vi "altera_atp_novo.vi"(0 "File Path Control":path=path "C:/Users/Flavio-CPGEI/Documents/ATPdata/work/Sistema_COELBA_2.atp", 5 "Condição de carga":string="0", 7 "Resistência de falta":string="0", 9 "Tipo de falta":string="0", 11 "Local de falta":string="0", 12 "Instante de falta (º)":string="0") -> (4 "path":path, 6 "Erro - chaves":bool, 8 "Erro - impedâncias":bool, 10 "Erro - string lenght":bool, 15 "error out":errorcluster)   [LabVIEW 2014]
panel:
  in  "SALVAR?":bool=TRUE
  out "substring":string
  out "index of element":i32
  out "tamanho final":i32
  out "Array inicial":i32[](array[numeric])
  out "tamanho inicial":i32
  out "Array final":i32[](array[numeric])
  out "Resistência de falta 2":string
  out "result string":string
  in  "Resistência":string="999"
  out "IMPEDÂNCIAS":string
  in  "Ciclo em falta":string="1"
  in  "atraso":dbl=0.001431
  out "CHAVES":string
  # "Saídas"
  # "Entradas ____________________________________________________________________________"
  # "carga_redebt"
  # "carga_delta"
  # "Condições padrão ___________________________________________________________________________________________________"
  # "Instante de falta"
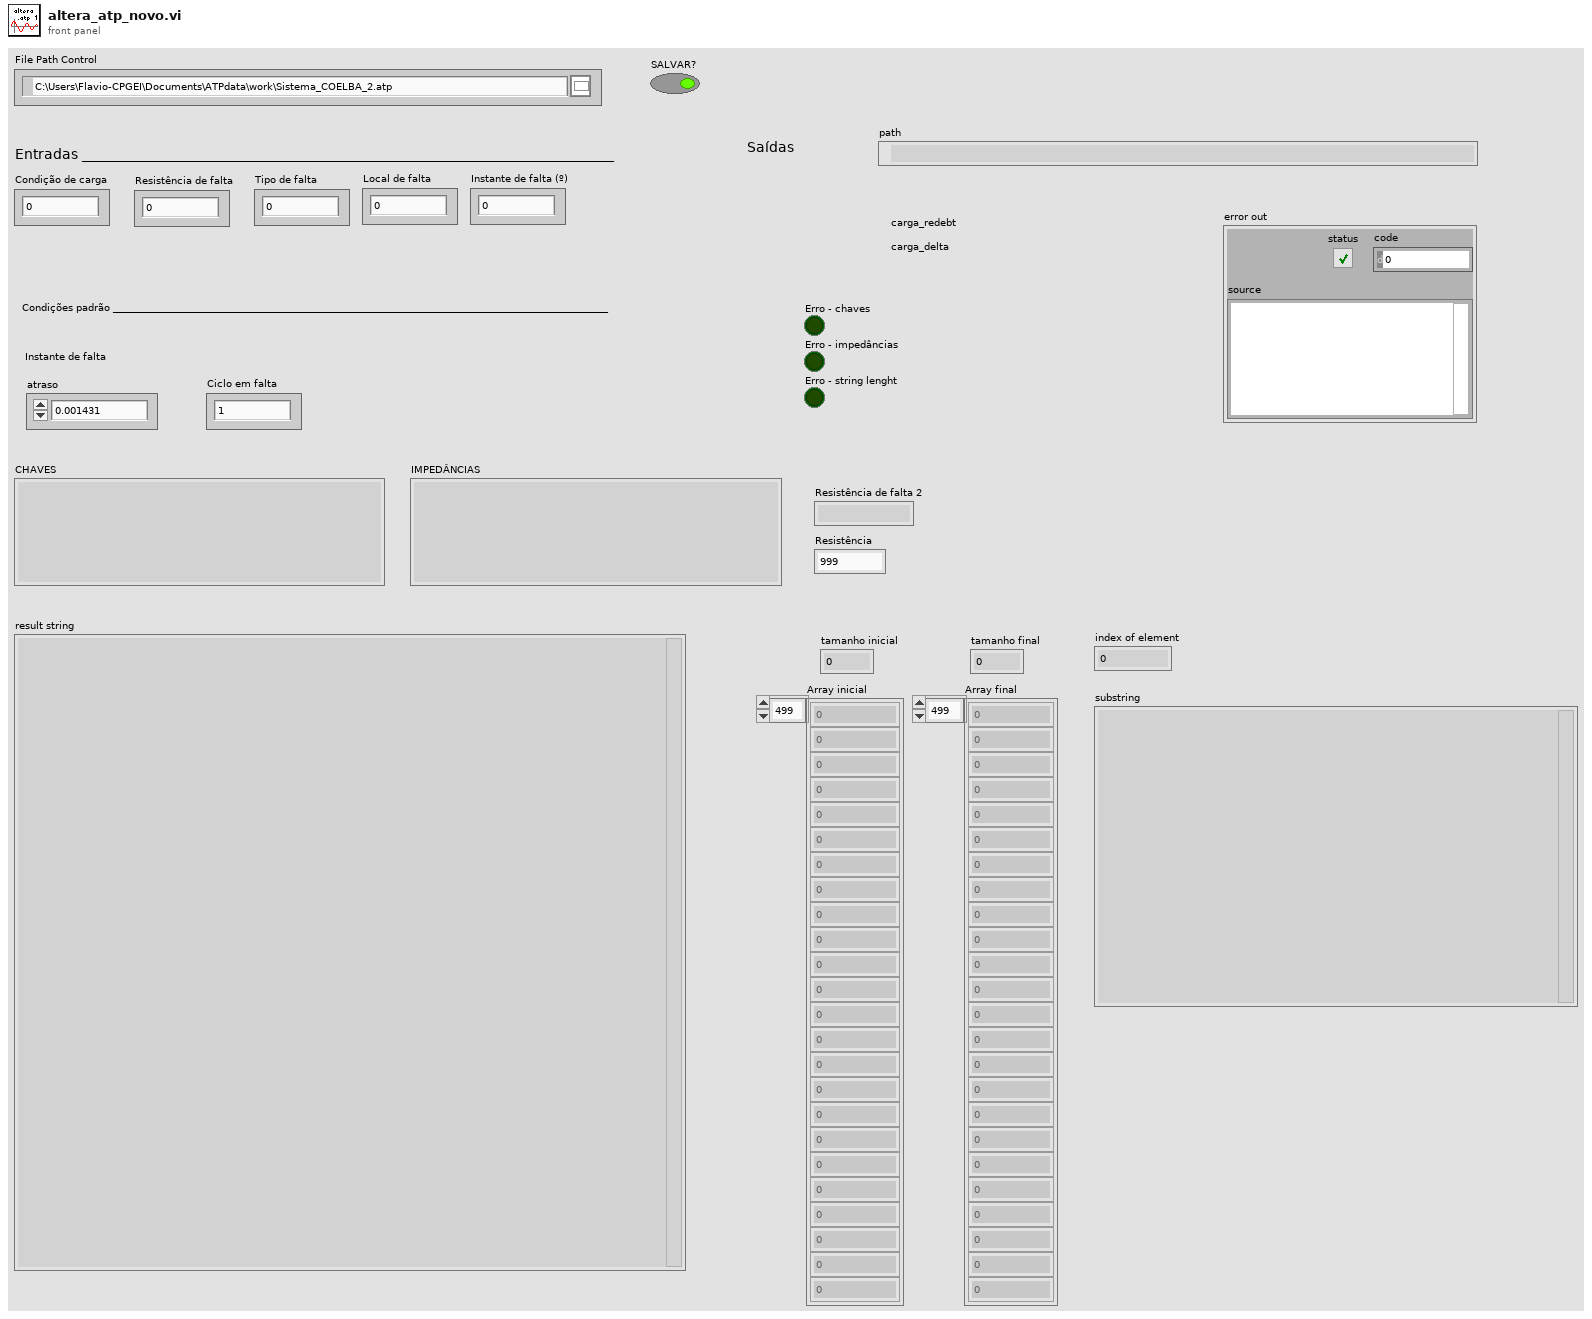
[diagram p1: front panel]
types:
  T1 = enum16{"open", "replace", "create", "open or create", "replace or create", "replace or create with confirmation"}
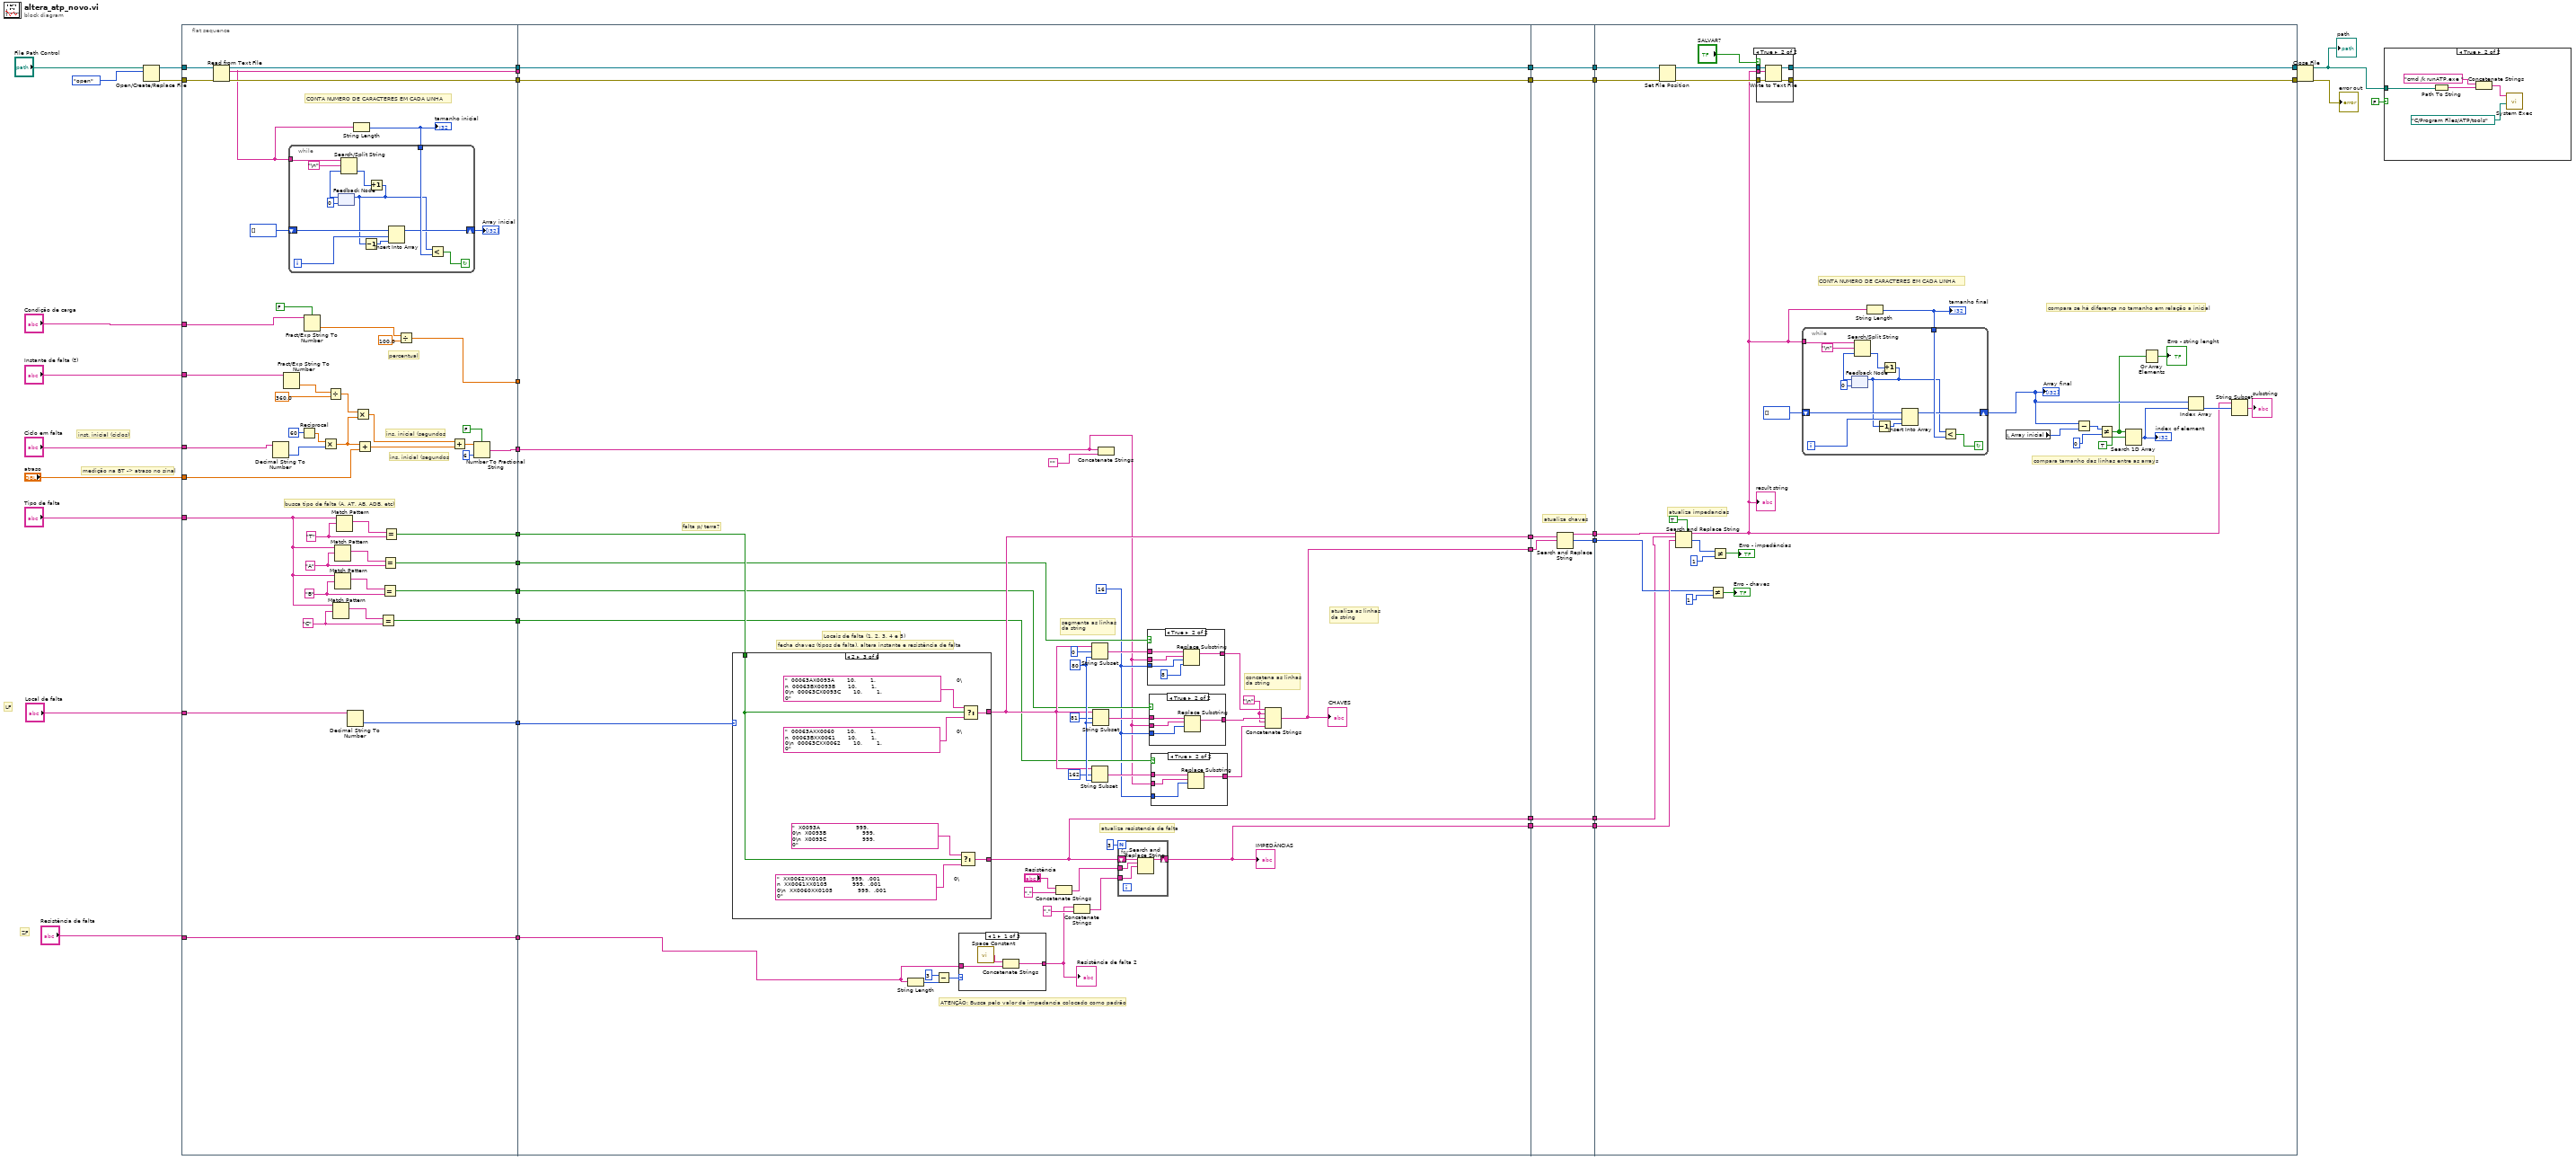
[diagram p0: block diagram]
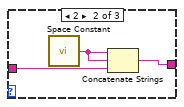
[diagram p3: hidden frame]
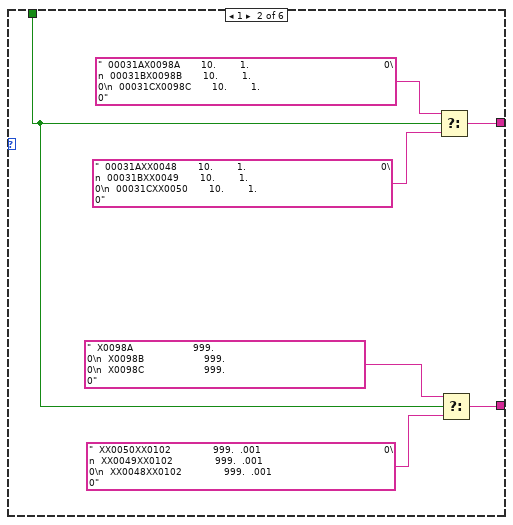
[diagram p9: hidden frame]
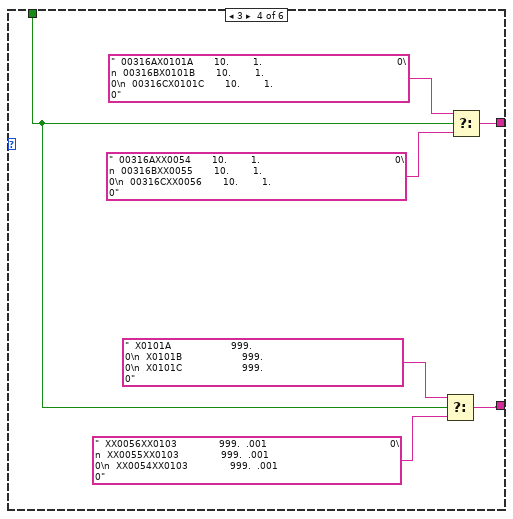
[diagram p10: hidden frame]
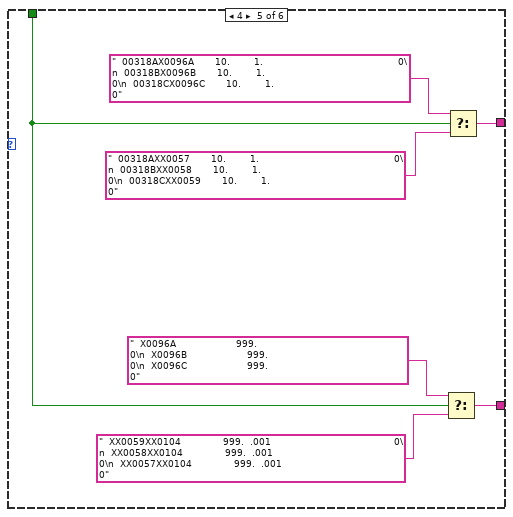
[diagram p11: hidden frame]
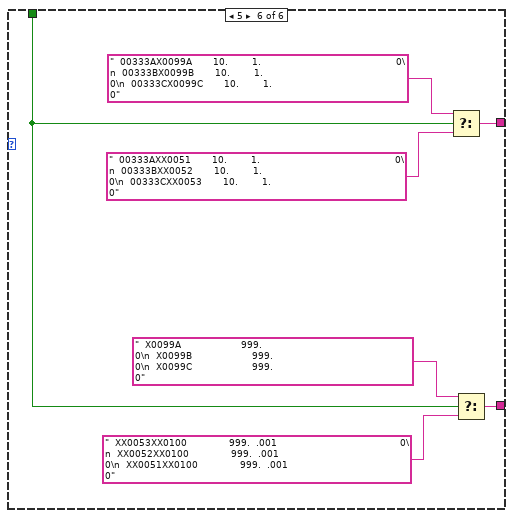
[diagram p12: hidden frame]
diagram:
  # "medição na BT -> atraso no sinal"
  # "inst. inicial (ciclos)"
  # "LF"
  # "TF"
  # "IF"
  # "ZF"
  n1 = Open/Create/Replace File(file path (use dialog)="File Path Control", operation (0:open)=T1."open") -> (refnum out=w20:refnum<file>, error out=w19:errorcluster)  [unwired: 4 in, 1 out]
  n2 = flat-sequence {
    tunnel: "Local de falta" -> [w84]
    tunnel: "Tipo de falta" -> [w70]
    tunnel: "Instante de falta (º)" -> [w66]
    tunnel: [w83] -> w39
    tunnel: [w80] -> w38
    tunnel: [w73] -> w37
    tunnel: [w72] -> w36
    tunnel: [w71] -> w35
    tunnel: [w58] -> w34
    tunnel: "Ciclo em falta" -> [w67]
    tunnel: "atraso" -> [w57]
    tunnel: [w54] -> w28
    tunnel: "Resistência de falta" -> [w54]
    tunnel: "Condição de carga" -> [w52]
    tunnel: [w45] -> w25
    tunnel: [w41] -> w24
    tunnel: [w51] -> w23
    tunnel: [w50] -> w22
    tunnel: w20 -> [w49]
    tunnel: w19 -> [w48]
    tunnel: w39 -> [w128]
    tunnel: w38 -> [w127]
    tunnel: w37 -> [w109]
    tunnel: w36 -> [w111]
    tunnel: w35 -> [w114]
    tunnel: [w115] -> w12
    tunnel: [w126] -> w11
    tunnel: w34 -> [w98]
    tunnel: w28 -> [w101]
    tunnel: w25 -> [_]
    tunnel: w24 -> [_]
    tunnel: w23 -> [w119]
    tunnel: [w119] -> w10
    tunnel: [w118] -> w8
    tunnel: w22 -> [w118]
    tunnel: [w117] -> w6
    tunnel: [w116] -> w4
    tunnel: w12 -> [w197]
    tunnel: w11 -> [w198]
    tunnel: w10 -> [w202]
    tunnel: [w202] -> w9
    tunnel: w8 -> [w201]
    tunnel: [w201] -> w7
    tunnel: w6 -> [w200]
    tunnel: [w200] -> w5
    tunnel: w4 -> [w199]
    tunnel: [w199] -> w3
    tunnel: [w196] -> w2
    tunnel: [w195] -> w1
    tunnel: w9 -> [w227]
    tunnel: w7 -> [w229]
    tunnel: [w232] -> w18
    tunnel: [w231] -> w17
    tunnel: w5 -> [w204]
    tunnel: w3 -> [w230]
    tunnel: w2 -> [w206]
    tunnel: w1 -> [w205]
    frame #0 {
      w74 = "C" ("regular expression")
      w76 = "B" ("regular expression")
      w78 = "A" ("regular expression")
      w81 = "T" ("regular expression")
      # "percentual"
      # "CONTA NUMERO DE CARACTERES EM CADA LINHA"
      # "busca tipo de falta (A, AT, AB, ADB, etc)"
      # "ins. inicial (segundos"
      # "ins. inicial (segundos"
      n3 = Read from Text File(file (use dialog)=w49, error in=w48) -> (refnum out=w51:refnum<file>, text=w41:string, error out=w50:errorcluster)  [unwired: 2 in, 1 out]
      n4 = Decimal String To Number(string=w67) -> (number=w68:i32)  [unwired: 2 in, 1 out]
      n5 = Fract/Exp String To Number(string=w66) -> (number=w64:dbl)  [unwired: 3 in, 1 out]
      n6 = Reciprocal(x=60) -> (1/x=w69:dbl)
      n7 = Fract/Exp String To Number(use system decimal point (T)=FALSE, string=w52) -> (number=w47:dbl)  [unwired: 2 in, 1 out]
      n8 = Multiply(x=w69, y=w68) -> (x*y=w65:dbl)
      n9 = Divide(x=w64, y=360.0) -> (x/y=w62:dbl)
      n10 = Match Pattern(string=w70, regular expression=w74) -> (match substring=w75:string)  [unwired: 1 in, 3 out]
      n11 = Match Pattern(string=w70, regular expression=w76) -> (match substring=w77:string)  [unwired: 1 in, 3 out]
      n12 = Match Pattern(string=w70, regular expression=w78) -> (match substring=w79:string)  [unwired: 1 in, 3 out]
      n13 = Match Pattern(string=w70, regular expression=w81) -> (match substring=w82:string)  [unwired: 1 in, 3 out]
      n14 = Decimal String To Number(string=w84) -> (number=w83:i32)  [unwired: 2 in, 1 out]
      n15 = String Length(string=w41) -> (length=w43:i32)
      "tamanho inicial" <- w43
      n16 = while {
        tunnel: w41 -> [w95]
        shift-right: [w87] -> w42
        shift-left: i32[] [] -> [w91]
        tunnel: w43 -> [w89]
        i -> [w90]
        stop <- w88 continue-if-true
        n17 = feedback #1(0) -> (w93:i32)
        n18 = Search/Split String(string=w95, search string/char (-)="\n", offset (0)=w93) -> (offset of match=w94:i32)  [unwired: 2 out]
        n19 = Increment(x=w94) -> (x+1=w85:i32)
        n20 = feedback-in #1(w85) -> ()
        n21 = Decrement(x=w85) -> (x-1=w86:i32)
        n22 = Insert Into Array(array=w91, index=w90, new element=w86) -> (w87:i32[])
        n23 = Less?(x=w85, y=w89) -> (x < y?=w88:bool)
      }
      "Array inicial" <- w42
      n24 = Multiply(x=w62, y=w65) -> (x*y=w60:dbl)
      n25 = Add(x=w65, y=w57) -> (x+y=w61:dbl)
      n26 = Equal?(x=w75, y=w74) -> (x = y?=w71:bool)
      n27 = Equal?(x=w77, y=w76) -> (x = y?=w72:bool)
      n28 = Equal?(x=w79, y=w78) -> (x = y?=w73:bool)
      n29 = Equal?(x=w82, y=w81) -> (x = y?=w80:bool)
      n30 = Divide(x=w47, y=100.0) -> (x/y=w45:dbl)
      n31 = Add(x=w60, y=w61) -> (x+y=w59:dbl)
      n32 = Number To Fractional String(use system decimal point (T)=FALSE, number=w59, precision (6)=i16 6) -> (F-format string=w58:string)  [unwired: 1 in]
    }
    frame #1 {
      w97 = "\n"
      w107 = 16 ("offset (0)")
      w132 = 80 ("length (rest)")
      # "ATENÇÃO: Busca pelo valor de impedancia colocado como padrão"
      # "atualiza resistencia de falta"
      # "concatena as linhas\nda string"
      # "atualiza as linhas\nda string"
      # "segmenta as linhas\nda string"
      # "fecha chaves (tipos de falta), altera instante e resistência de falta"
      # "falta p/ terra?"
      # "Locais de falta (1, 2, 3, 4 e 5)"
      n33 = case shown="2" w128 {
        tunnel: [_ w164 w171 w178 w185 w193] -> w115
        tunnel: w127 -> [_ w161 w167 w174 w181 w188]
        tunnel: [_ w160 w168 w175 w182 w189] -> w117
        frame Default {
        }
        frame 1 {
          n34 = Select(t="  00031AX0098A       10.        1.                                             0\n  00031BX0098B       10.        1.                                             0\n  00031CX0098C       10.        1.                                             0" ("search string"), s=w161, f="  00031AXX0048       10.        1.                                             0\n  00031BXX0049       10.        1.                                             0\n  00031CXX0050       10.        1.                                             0" ("search string")) -> (s? t:f=w164:string)
          n35 = Select(t="  X0098A                    999.                                               0\n  X0098B                    999.                                               0\n  X0098C                    999.                                               0" ("search string"), s=w161, f="  XX0050XX0102              999.  .001                                         0\n  XX0049XX0102              999.  .001                                         0\n  XX0048XX0102              999.  .001                                         0" ("search string")) -> (s? t:f=w160:string)
        }
        frame 2 {
          n36 = Select(t="  X0093A                    999.                                               0\n  X0093B                    999.                                               0\n  X0093C                    999.                                               0" ("search string"), s=w167, f="  XX0062XX0105              999.  .001                                         0\n  XX0061XX0105              999.  .001                                         0\n  XX0060XX0105              999.  .001                                         0" ("search string")) -> (s? t:f=w168:string)
          n37 = Select(t="  00063AX0093A       10.        1.                                             0\n  00063BX0093B       10.        1.                                             0\n  00063CX0093C       10.        1.                                             0" ("search string"), s=w167, f="  00063AXX0060       10.        1.                                             0\n  00063BXX0061       10.        1.                                             0\n  00063CXX0062       10.        1.                                             0" ("search string")) -> (s? t:f=w171:string)
        }
        frame 3 {
          n38 = Select(t="  X0101A                    999.                                               0\n  X0101B                    999.                                               0\n  X0101C                    999.                                               0" ("search string"), s=w174, f="  XX0056XX0103              999.  .001                                         0\n  XX0055XX0103              999.  .001                                         0\n  XX0054XX0103              999.  .001                                         0" ("search string")) -> (s? t:f=w175:string)
          n39 = Select(t="  00316AX0101A       10.        1.                                             0\n  00316BX0101B       10.        1.                                             0\n  00316CX0101C       10.        1.                                             0" ("search string"), s=w174, f="  00316AXX0054       10.        1.                                             0\n  00316BXX0055       10.        1.                                             0\n  00316CXX0056       10.        1.                                             0" ("search string")) -> (s? t:f=w178:string)
        }
        frame 4 {
          n40 = Select(t="  X0096A                    999.                                               0\n  X0096B                    999.                                               0\n  X0096C                    999.                                               0" ("search string"), s=w181, f="  XX0059XX0104              999.  .001                                         0\n  XX0058XX0104              999.  .001                                         0\n  XX0057XX0104              999.  .001                                         0" ("search string")) -> (s? t:f=w182:string)
          n41 = Select(t="  00318AX0096A       10.        1.                                             0\n  00318BX0096B       10.        1.                                             0\n  00318CX0096C       10.        1.                                             0" ("search string"), s=w181, f="  00318AXX0057       10.        1.                                             0\n  00318BXX0058       10.        1.                                             0\n  00318CXX0059       10.        1.                                             0" ("search string")) -> (s? t:f=w185:string)
        }
        frame 5 {
          n42 = Select(t="  00333AX0099A       10.        1.                                             0\n  00333BX0099B       10.        1.                                             0\n  00333CX0099C       10.        1.                                             0" ("search string"), s=w188, f="  00333AXX0051       10.        1.                                             0\n  00333BXX0052       10.        1.                                             0\n  00333CXX0053       10.        1.                                             0" ("search string")) -> (s? t:f=w193:string)
          n43 = Select(t="  X0099A                    999.                                               0\n  X0099B                    999.                                               0\n  X0099C                    999.                                               0" ("search string"), s=w188, f="  XX0053XX0100              999.  .001                                         0\n  XX0052XX0100              999.  .001                                         0\n  XX0051XX0100              999.  .001                                         0" ("search string")) -> (s? t:f=w189:string)
        }
      }
      n44 = String Length(string=w101) -> (length=w104:i32)
      n45 = Subtract(x=3, y=w104) -> (x-y=w102:i32)
      n46 = case shown="1" w102 {
        tunnel: w101 -> [w135 w138 w139]
        tunnel: [w134 w137 w139] -> w100
        frame 1 {
          n47 = call <vilib>:"Space Constant.vi"() -> ("String"=w133:string)
          n48 = Concatenate Strings(w133, w135) -> (w134:string)
        }
        frame 2 {
          n49 = call <vilib>:"Space Constant.vi"() -> ("String"=w136:string)
          n50 = Concatenate Strings(w136, w136, w138) -> (w137:string)
        }
        frame Default {
        }
      }
      "Resistência de falta 2" <- w100
      n51 = Concatenate Strings("Resistência", ".") -> (w120:string)
      n52 = Concatenate Strings(w100, ".") -> (w123:string)
      n53 = String Subset(string=w115, offset (0)=162, length (rest)=w132) -> (substring=w113:string)
      n54 = String Subset(string=w115, offset (0)=0, length (rest)=w132) -> (substring=w108:string)
      n55 = String Subset(string=w115, offset (0)=81, length (rest)=w132) -> (substring=w110:string)
      n56 = Concatenate Strings(w98, "") -> ()  [unwired: 1 out]
      n57 = for {
        N: 3 -> [_]
        tunnel: w120 -> [w158]
        shift-right: [w157] -> w116
        shift-left: w117 -> [w159]
        tunnel: w123 -> [w156]
        n58 = Search and Replace String(input string=w159, search string=w158, replace string=w156) -> (result string=w157:string)  [unwired: 5 in, 3 out]
      }
      "IMPEDÂNCIAS" <- w116
      n59 = case shown="True" w109 {
        tunnel: w108 -> [w140 w145]
        tunnel: [w140 w144] -> w106
        tunnel: w98 -> [_ w143]
        tunnel: w107 -> [_ w142]
        frame False {
        }
        frame True {
          n60 = Replace Substring(2:8 ("length (len. of substring)"), 3:w142, 4:w143, 5:w145) -> (1:w144:string)  [unwired: 1 out]
        }
      }
      n61 = case shown="True" w111 {
        tunnel: w110 -> [w146 w150]
        tunnel: [w146 w149] -> w105
        tunnel: w98 -> [_ w148]
        tunnel: w107 -> [_ w147]
        frame False {
        }
        frame True {
          n62 = Replace Substring(3:w147, 4:w148, 5:w150) -> (1:w149:string)  [unwired: 1 in, 1 out]
        }
      }
      n63 = case shown="True" w114 {
        tunnel: w113 -> [w151 w155]
        tunnel: [w151 w154] -> w112
        tunnel: w98 -> [_ w153]
        tunnel: w107 -> [_ w152]
        frame False {
        }
        frame True {
          n64 = Replace Substring(3:w152, 4:w153, 5:w155) -> (1:w154:string)  [unwired: 1 in, 1 out]
        }
      }
      n65 = Concatenate Strings(w106, w97, w105, w97, w112) -> (w126:string)
      "CHAVES" <- w126
    }
    frame #2 {
      # "atualiza chaves"
      n66 = Search and Replace String(search string=w197, replace string=w198) -> (result string=w196:string, number of replacements=w195:i32)  [unwired: 6 in, 2 out]
    }
    frame #3 {
      # "compara se há diferença no tamanho em relação a inicial"
      # "compara tamanho das linhas entre as arrays"
      # "CONTA NUMERO DE CARACTERES EM CADA LINHA"
      # "atualiza impedancias"
      n67 = Set File Position(refnum=w227, error in=w229) -> (refnum out=w226:refnum<file>, error out=w228:errorcluster)  [unwired: 2 in]
      n68 = Search and Replace String(multiline?=TRUE ("multiline? (F)"), input string=w206, search string=w204, replace string=w230) -> (result string=w210:string, number of replacements=w222:i32)  [unwired: 4 in, 2 out]
      "result string" <- w210
      n69 = Not Equal?(x=w205, y=1) -> (x != y?=→"Erro - chaves":bool)
      n70 = Not Equal?(x=w222, y=1) -> (x != y?=→"Erro - impedâncias":bool)
      n71 = case shown="True" "SALVAR?" {
        tunnel: [w245 w251] -> w232
        tunnel: [w246 w250] -> w231
        tunnel: w210 -> [_ w249]
        tunnel: w228 -> [w245 w248]
        tunnel: w226 -> [w246 w247]
        frame False {
        }
        frame True {
          n72 = Write to Text File(file (use dialog)=w247, text=w249, error in=w248) -> (refnum out=w250:refnum<file>, error out=w251:errorcluster)  [unwired: 1 in, 1 out]
        }
      }
      n73 = String Length(string=w210) -> (length=w223:i32)
      "tamanho final" <- w223
      n74 = while {
        tunnel: w210 -> [w243]
        shift-right: [w235] -> w212
        shift-left: i32[] [] -> [w239]
        tunnel: w223 -> [w237]
        i -> [w238]
        stop <- w236 continue-if-true
        n75 = feedback #2(0) -> (w241:i32)
        n76 = Search/Split String(string=w243, search string/char (-)="\n", offset (0)=w241) -> (offset of match=w242:i32)  [unwired: 2 out]
        n77 = Increment(x=w242) -> (x+1=w233:i32)
        n78 = feedback-in #2(w233) -> ()
        n79 = Decrement(x=w233) -> (x-1=w234:i32)
        n80 = Insert Into Array(array=w239, index=w238, new element=w234) -> (w235:i32[])
        n81 = Less?(x=w233, y=w237) -> (x < y?=w236:bool)
      }
      "Array final" <- w212
      n82 = local read "Array inicial"() -> (w217:i32[])
      n83 = Subtract(x=w212, y=w217) -> (x-y=w215:i32[])
      n84 = Not Equal?(x=w215, y=0) -> (x != y?=w208:bool[])
      n85 = Search 1D Array(1D array=w208, element=TRUE) -> (index of element=w213:i32)  [unwired: 1 in]
      "index of element" <- w213
      n86 = Or Array Elements(Boolean array=w208) -> (logical OR=→"Erro - string lenght":bool)
      n87 = Index Array(array=w212, index=w213) -> (element=w211:i32)
      n88 = String Subset(string=w210, offset (0)=w211) -> (substring=→"substring":string)  [unwired: 1 in]
    }
  }
  n89 = Close File(refnum=w17, error in=w18) -> (path=w14:path, error out=→"error out":errorcluster)
  "path" <- w14
  n90 = case shown="True" FALSE {
    tunnel: w14 -> [_ w252]
    frame False {
    }
    frame True {
      n91 = Path To String(path=w252) -> (string=w255:string)
      n92 = Concatenate Strings("cmd /k runATP.exe " ("string"), w255) -> (w253:string)
      n93 = call <vilib>:"System Exec.vi"("working directory"=path "C:/Program Files/ATP/tools", "command line"=w253) -> ()  [unwired: 6 in, 4 out]
    }
  }
